vi "Dialog (Dynamic).vi"(4 "Open if error? [T]":bool=TRUE, 6 "Open if no error? [F]":bool, 7 "Dynamic? [T]":bool=TRUE, 8 "error in (no error)":errorcluster) -> (0 "error out":errorcluster)   [LabVIEW 2020, in "Multiple Errors.lvclass"]
doc: "Indicates whether an error occurred. If an error occurred, this VI returns a description of the error and optionally displays a dialog box."
uses:
  Multiple Errors.lvclass
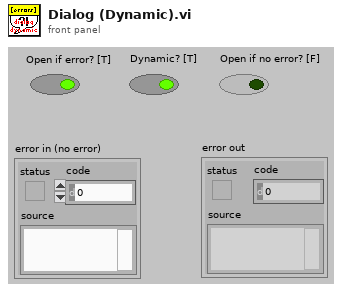
[diagram p1: front panel]
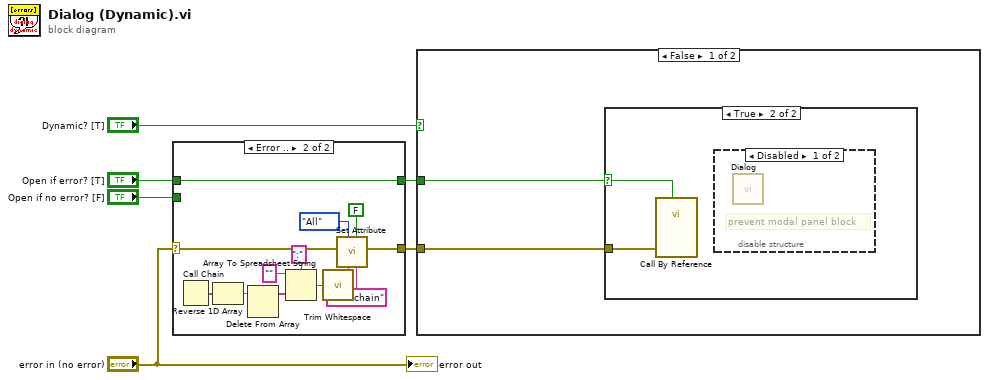
[diagram p0: block diagram]
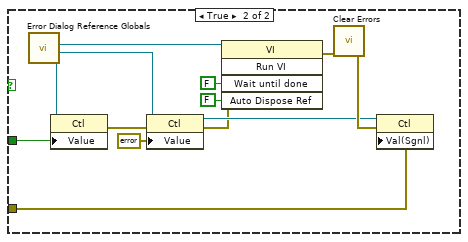
[diagram p5: hidden frame]
diagram:
  n1 = case shown="Error .." "error in (no error)" {
    selector: "error in (no error)" -> [w8 w13]
    tunnel: [w8 w12] -> w4
    tunnel: "Open if error? [T]" -> [_ w9]
    tunnel: [w7 w9] -> w2
    tunnel: "Open if no error? [F]" -> [w7 _]
    frame No Error {
    }
    frame Error {
      n2 = Call Chain() -> (call chain=w16:string[])
      n3 = Reverse 1D Array(array=w16) -> (reversed array=w14:string[])
      n4 = Delete From Array(array=w14) -> (array with subset deleted=w15:string[])  [unwired: 2 in, 1 out]
      n5 = Array To Spreadsheet String(delimiter (Tab)=":", array=w15, 3:"" ("format string")) -> (spreadsheet string=w17:string)
      n6 = call <vilib>:"Trim Whitespace.vi"("string"=w17) -> ("trimmed string"=w18:string)  [unwired: 1 in]
      n7 = call "Set Attribute.vi"("Attribute [\"Info\"]"="Call chain" ("Attribute [\"Info\"]"), "Overwrite? [T]"=FALSE, "Text"=w18, "Error [Last]"=enum16{"First", "Last", "All"}."All", "error in (no error)"=w13) -> ("error out"=w12:errorcluster)  [unwired: 6 in]
    }
  }
  n8 = case shown="False" "Dynamic? [T]" {
    tunnel: w4 -> [w23 w31]
    tunnel: w2 -> [w22 w27]
    frame False {
      n9 = case shown="True" w22 {
        selector: w22 -> [_ w24]
        tunnel: w23 -> [_ w25]
        frame False {
        }
        frame True {
          n10 = call-by-ref "?"("Open? [T]"=w24, "error in (no error)"=w25) -> ()  [unwired: 12 in, 2 out]
          n11 = disable-structure shown="Disabled" {
            frame Disabled {
              # "prevent modal panel block"
              n12 = call "Dialog.vi"() -> ()  [unwired: 12 in]
            }
            frame Enabled {
            }
          }
        }
      }
    }
    frame True {
      n13 = call "Error Dialog Reference Globals.vi"() -> ("Open?"=w28:refnum<vi>, "Error in"=w34:refnum<vi>, "VI reference"=w29:refnum<vi>)  [unwired: 9 in]
      n14 = property class="Ctl"(reference=w28, "Value"=w27) -> (error out=w26:errorcluster)  [unwired: 1 in, 1 out]
      n15 = property class="Ctl"(reference=w34, error in=w26, "Value"=errorcluster {"status"=FALSE, "code"=0, "source"=""} ("error in (no error)")) -> (reference out=w33:refnum<vi>, error out=w30:errorcluster)
      n16 = invoke class="VI" method="Run VI"(reference=w29, error in=w30, "Wait until done"=FALSE ("Wait Until Done"), "Auto Dispose Ref"=FALSE ("Auto Dispose Reference")) -> (error out=w36:errorcluster)  [unwired: 1 in, 4 out]
      n17 = call <vilib>:"Clear Errors.vi"("error in (no error)"=w36) -> ("error out"=w35:errorcluster)  [unwired: 5 in, 1 out]
      n18 = property class="Ctl"(reference=w33, error in=w35, "Val(Sgnl)"=w31) -> ()  [unwired: 2 out]
    }
  }
  "error out" <- "error in (no error)"
